vi "Stop Core.vi"(10 "final error code":i32, 11 "[M] TDMS Save in":refnum<class "[M] TDMS Save.lvclass">) -> (3 "[M] TDMS Save out":refnum<class "[M] TDMS Save.lvclass">)   [LabVIEW 2023, in "[M] TDMS Save.lvlib" / "[M] TDMS Save.lvclass"]
doc: "(<B>Filename</B>: Actor Framework.lvlib:Actor.lvclass:Stop Core.vi)\n\nDefines what the actor does before it stops. Use the <B>final error code</B> input to determine whether the actor shut down in response to an error.\n\nBy default, this method passes the Stop message along to all auto-stop nested actors. A descendant class may override this method to define additional behavior, such as shutting down any processes the actor initiated in its override of the Actor Core method."
uses:
  [M] TDMS Save.lvclass
  [M] TDMS Save.lvclass/[M] TDMS Save.ctl
  <vilib>/ActorFramework/Actor/Actor.lvclass
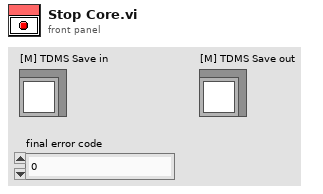
[diagram p1: front panel]
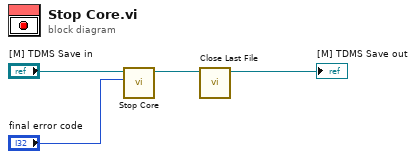
[diagram p0: block diagram]
diagram:
  n1 = call-parent "Stop Core.vi"("final error code"="final error code", "Actor in"="[M] TDMS Save in") -> ("Actor out"=w2:refnum<class "[M] TDMS Save.lvclass">)  [unwired: 9 in]
  n2 = call "Close Last File.vi"("[M] TDMS Save in"=w2) -> ("[M] TDMS Save out"=→"[M] TDMS Save out":refnum<class "[M] TDMS Save.lvclass">)  [unwired: 9 in, 1 out]
